vi "Remove Async Message from Map.vi"(8 "error in (no error)":errorcluster, 10 "Message":refnum<class "Async Message.lvclass">, 11 "Async Methods Actor in":refnum<class "Async Methods Actor.lvclass">) -> (0 "error out":errorcluster, 3 "Async Methods Actor out":refnum<class "Async Methods Actor.lvclass">)   [LabVIEW 2021, in "Async Methods Actor.lvlib" / "Async Methods Actor.lvclass"]
uses:
  Async Methods Actor.lvclass
  Async Methods Actor.lvclass/Async Methods Actor.ctl
  Write Async Message Execution Status Map.vi
  Write Async Message Execution Status Map.vi/3adbf29e-89d7-4ecb-a2bd-8a8b89d527f8.vi
  Async Methods Actor Messages/Async Message/Async Message.lvclass
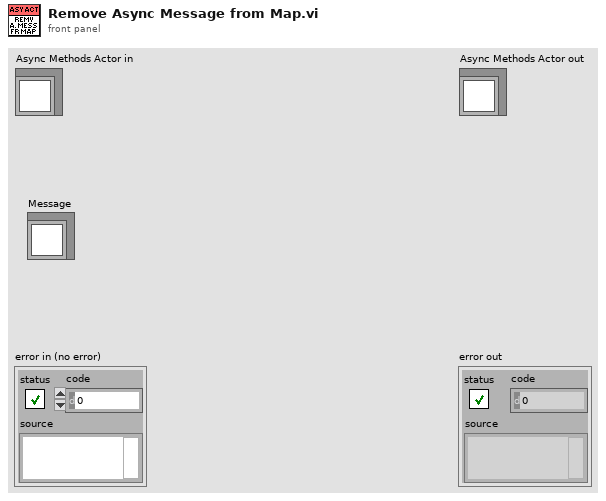
[diagram p1: front panel]
types:
  T1 = typedef "Async Methods Actor.lvlib/Async Methods Actor.lvclass/Async Message Execution Status Map.ctl" = map{string, T2}
  T2 = typedef "Async Methods Actor.lvlib/Async Methods Actor.lvclass/Async Message Execution Status.ctl" = cluster{"C&C Clones Running":u32, "C&F Clones Launched":u32, "GUID":string}
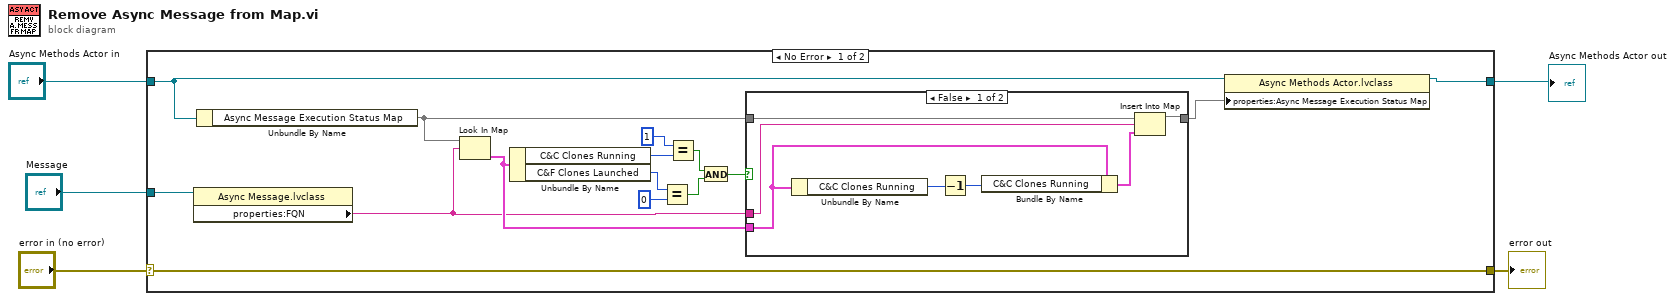
[diagram p0: block diagram]
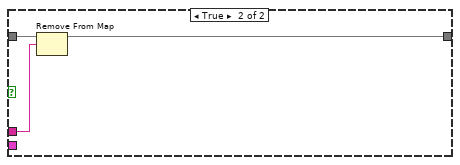
[diagram p2: hidden frame]
diagram:
  n1 = case shown="No Error" "error in (no error)" {
    selector: "error in (no error)" -> [w20 w32]
    tunnel: [w20 w32] -> w4
    tunnel: [w9 w31] -> w2
    tunnel: "Async Methods Actor in" -> [w10 w31]
    tunnel: "Message" -> [w7 _]
    frame No Error {
      n2 = property class="Async Message.lvclass"(reference=w7) -> ("properties:FQN"=w6:string)  [unwired: 1 in, 2 out]
      n3 = Unbundle By Name(w10) -> ("Async Message Execution Status Map"=w19:T1)
      n4 = Look In Map(map=w19, key=w6) -> (value=w11:T2)  [unwired: 1 in, 1 out]
      n5 = Unbundle By Name(w11) -> ("C&C Clones Running"=w18:u32, "C&F Clones Launched"=w16:u32)
      n6 = Equal?(x=w16, y=u32 0) -> (x = y?=w13:bool)
      n7 = Equal?(x=u32 1 ("y"), y=w18) -> (x = y?=w14:bool)
      n8 = And(x=w14, y=w13) -> (x .and. y?=w12:bool)
      n9 = case shown="False" w12 {
        tunnel: w19 -> [w24 w29]
        tunnel: [w22 w30] -> w8
        tunnel: w11 -> [w23 _]
        tunnel: w6 -> [w21 w28]
        frame False {
          n10 = Unbundle By Name(w23) -> ("C&C Clones Running"=w26:u32)
          n11 = Decrement(x=w26) -> (x-1=w27:u32)
          n12 = Bundle By Name(cluster=w23, "C&C Clones Running"=w27) -> (w25:T2)
          n13 = Insert Into Map(map in=w24, key=w21, value=w25) -> (map out=w22:T1)  [unwired: 2 out]
        }
        frame True {
          n14 = Remove From Map(10:w28, 11:w29) -> (3:w30:T1)  [unwired: 2 out]
        }
      }
      n15 = property class="Async Methods Actor.lvclass"(reference=w10, "properties:Async Message Execution Status Map"=w8) -> (reference out=w9:refnum<class "Async Methods Actor.lvclass">)  [unwired: 1 in, 1 out]
    }
    frame Error {
    }
  }
  "error out" <- w4
  "Async Methods Actor out" <- w2
